vi "SetBDClassCluster.vi"(8 "error in (no error)":errorcluster, 11 "BaseDevice.lvclass":refnum<class "BaseDevice.lvclass">) -> (0 "error out":errorcluster, 2 "BaseDev Data":T1={"Nom de ressource VISA"="", "DeviceCtrl"=[], "DataNames"=[], "ScanParamOut"=0.0, "HeaderString"="", "Functions"=[], "ScanFuncInd"=0, "Function"="", "StartStatPanel"=FALSE, "PanelVIRef"=refnum, "SubPanelRef"=refnum, "SubPanelCtrl"=[], "LoadedPanelIndex"=-1, "InstrumentName"="", "AvailFuncPan"=["ClassPanel"], "ScanTable"=[], "ScanPanelRef"=refnum, "ScanPanelPath"=path "", "Beforewait(ms)"=0, "Afterwait(ms)"=0, "SynchToClk(ms)"=-1, "FuncPanelIndex"=-1, "ClassQueue"=refnum, "ClassEvent"=refnum, "InstrParam"=[], "DatDisplayNm"=[], "ShowInstrNm"=[], "ShowParSuffix"=[], "ShowScanSuffix"=[], "ShowParValue"=[], "ParSuffix"=[], "ScanSuffix"=[], "Delta Time(ms)"=0, "BaseDataPath"=path "", "SubDatDisplayNm"=[], "SubScanTable(y)"=[], "SubVarParNm X"=[], "SubVarParNm Y"=[], "DataBindCtrl"=[], "DataCtrl"=[], "ReuseVarPar"=FALSE, "LastScanPos"=[], "BackForth"=FALSE, "ArrayDatNm"=[], "ArrayDisplNm"=[]}, 3 "BaseDevice.lvclass Out":refnum<class "BaseDevice.lvclass">)   [LabVIEW 2019, in "BaseDevice.lvclass"]
uses:
  BaseDevice.lvclass
  BDClassCluster.ctl
  BaseDevice.lvclass/BaseDevice.ctl
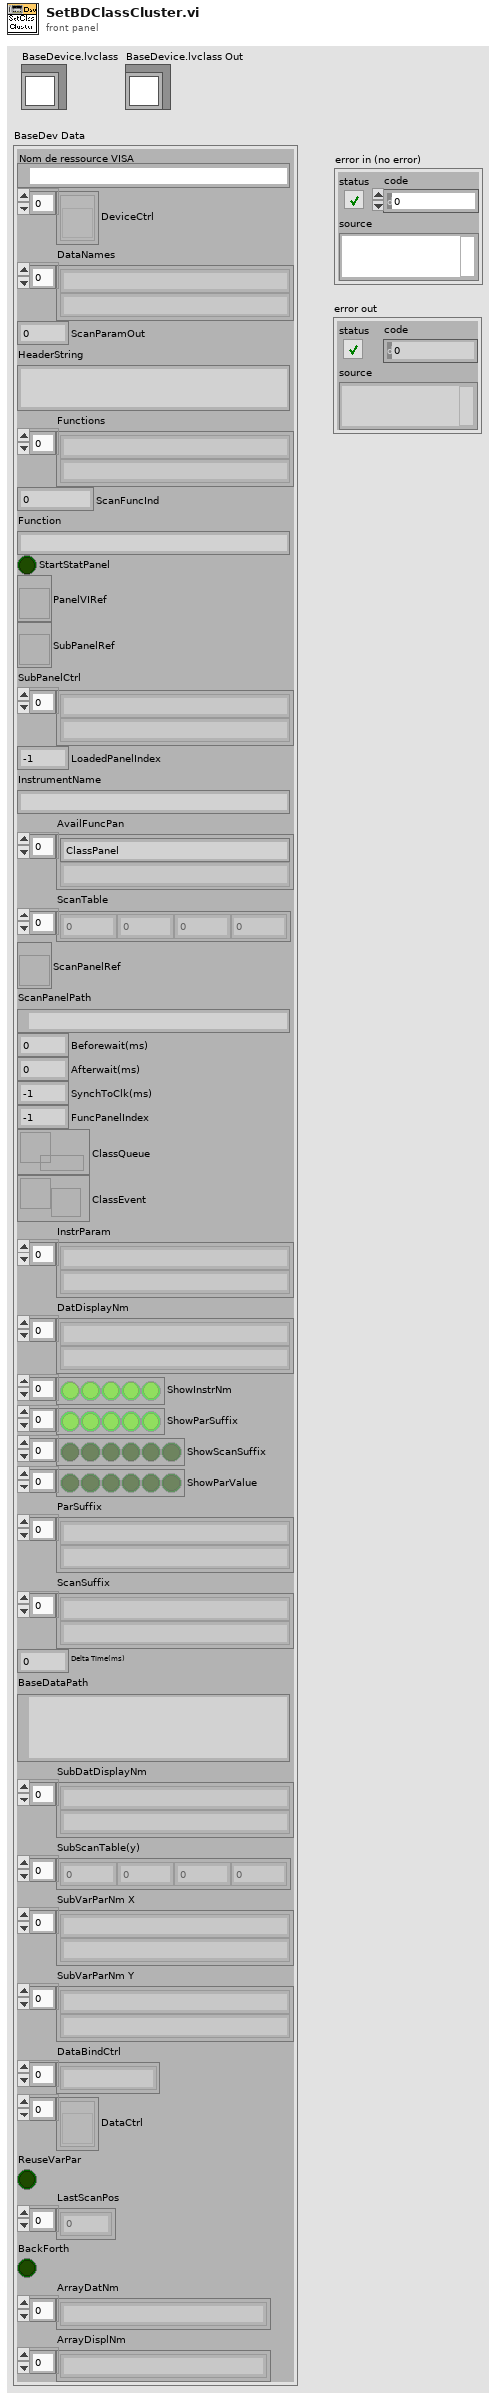
[diagram p1: front panel]
types:
  T1 = typedef "BDClassCluster.ctl" = cluster{"Nom de ressource VISA":refnum<visa-resource-name>, "DeviceCtrl":refnum<vi>[], "DataNames":string[], "ScanParamOut":dbl, "HeaderString":string, "Functions":string[], "ScanFuncInd":i32, "Function":string, "StartStatPanel":bool, "PanelVIRef":refnum<vi>, "SubPanelRef":refnum<vi>, "SubPanelCtrl":string[], "LoadedPanelIndex":i32, "InstrumentName":string, "AvailFuncPan":string[], "ScanTable":dbl[], "ScanPanelRef":refnum<vi>, "ScanPanelPath":path, "Beforewait(ms)":u32, "Afterwait(ms)":u32, "SynchToClk(ms)":i32, "FuncPanelIndex":i32, "ClassQueue":refnum<queue>, "ClassEvent":refnum<user-event>, "InstrParam":string[], "DatDisplayNm":string[], "ShowInstrNm":bool[], "ShowParSuffix":bool[], "ShowScanSuffix":bool[], "ShowParValue":bool[], "ParSuffix":string[], "ScanSuffix":string[], "Delta Time(ms)":u32, "BaseDataPath":path, "SubDatDisplayNm":string[], "SubScanTable(y)":dbl[], "SubVarParNm X":string[], "SubVarParNm Y":string[], "DataBindCtrl":string[], "DataCtrl":refnum<vi>[], "ReuseVarPar":bool, "LastScanPos":dbl[], "BackForth":bool, "ArrayDatNm":string[], "ArrayDisplNm":string[]}
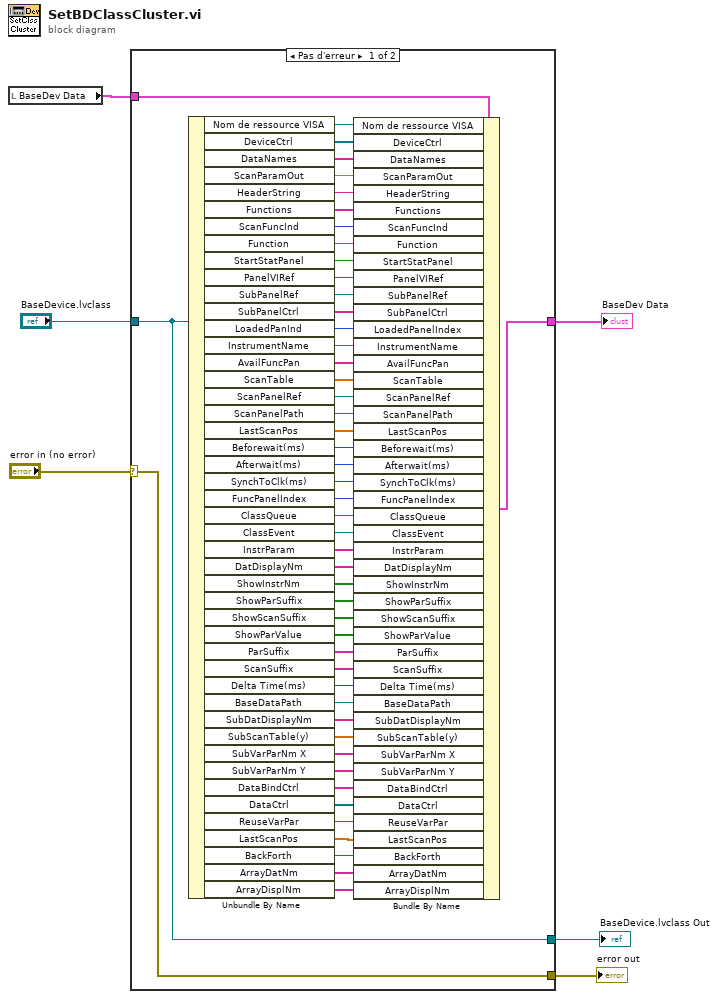
[diagram p0: block diagram]
diagram:
  n1 = local read "BaseDev Data"() -> (w2:T1)
  n2 = case shown="Pas d'erreur" "error in (no error)" {
    selector: "error in (no error)" -> [w56 w58]
    tunnel: "BaseDevice.lvclass" -> [w54 w59]
    tunnel: [w21 w57] -> w1
    tunnel: [w56 w58] -> w4
    tunnel: [w54 w59] -> w3
    tunnel: w2 -> [w55 w57]
    frame No Error {
      n3 = Unbundle By Name(w54) -> ("Nom de ressource VISA"=w53:refnum<visa-resource-name>, "DeviceCtrl"=w52:refnum<vi>[], "DataNames"=w51:string[], "ScanParamOut"=w50:dbl, "HeaderString"=w49:string, "Functions"=w48:string[], "ScanFuncInd"=w47:i32, "Function"=w46:string, "StartStatPanel"=w45:bool, "PanelVIRef"=w44:refnum<vi>, "SubPanelRef"=w43:refnum<vi>, "SubPanelCtrl"=w42:string[], "LoadedPanInd"=w41:i32, "InstrumentName"=w40:string, "AvailFuncPan"=w39:string[], "ScanTable"=w38:dbl[], "ScanPanelRef"=w22:refnum<vi>, "ScanPanelPath"=w23:path, "LastScanPos"=w14:dbl[], "Beforewait(ms)"=w24:u32, "Afterwait(ms)"=w25:u32, "SynchToClk(ms)"=w26:i32, "FuncPanelIndex"=w27:i32, "ClassQueue"=w28:refnum<queue>, "ClassEvent"=w29:refnum<user-event>, "InstrParam"=w30:string[], "DatDisplayNm"=w31:string[], "ShowInstrNm"=w32:bool[], "ShowParSuffix"=w33:bool[], "ShowScanSuffix"=w34:bool[], "ShowParValue"=w35:bool[], "ParSuffix"=w36:string[], "ScanSuffix"=w37:string[], "Delta Time(ms)"=w15:u32, "BaseDataPath"=w16:path, "SubDatDisplayNm"=w17:string[], "SubScanTable(y)"=w18:dbl[], "SubVarParNm X"=w19:string[], "SubVarParNm Y"=w20:string[], "DataBindCtrl"=w13:string[], "DataCtrl"=w12:refnum<vi>[], "ReuseVarPar"=w11:bool, "LastScanPos"=w10:dbl[], "BackForth"=w9:bool, "ArrayDatNm"=w8:string[], "ArrayDisplNm"=w7:string[])
      n4 = Bundle By Name(cluster=w55, "Nom de ressource VISA"=w53, "DeviceCtrl"=w52, "DataNames"=w51, "ScanParamOut"=w50, "HeaderString"=w49, "Functions"=w48, "ScanFuncInd"=w47, "Function"=w46, "StartStatPanel"=w45, "PanelVIRef"=w44, "SubPanelRef"=w43, "SubPanelCtrl"=w42, "LoadedPanelIndex"=w41, "InstrumentName"=w40, "AvailFuncPan"=w39, "ScanTable"=w38, "ScanPanelRef"=w22, "ScanPanelPath"=w23, "LastScanPos"=w14, "Beforewait(ms)"=w24, "Afterwait(ms)"=w25, "SynchToClk(ms)"=w26, "FuncPanelIndex"=w27, "ClassQueue"=w28, "ClassEvent"=w29, "InstrParam"=w30, "DatDisplayNm"=w31, "ShowInstrNm"=w32, "ShowParSuffix"=w33, "ShowScanSuffix"=w34, "ShowParValue"=w35, "ParSuffix"=w36, "ScanSuffix"=w37, "Delta Time(ms)"=w15, "BaseDataPath"=w16, "SubDatDisplayNm"=w17, "SubScanTable(y)"=w18, "SubVarParNm X"=w19, "SubVarParNm Y"=w20, "DataBindCtrl"=w13, "DataCtrl"=w12, "ReuseVarPar"=w11, "LastScanPos"=w10, "BackForth"=w9, "ArrayDatNm"=w8, "ArrayDisplNm"=w7) -> (w21:T1)
    }
    frame Error {
    }
  }
  "BaseDevice.lvclass Out" <- w3
  "error out" <- w4
  "BaseDev Data" <- w1
